vi "Privet.vi"(0 "imya":string) -> ()   [LabVIEW 2016]
uses:
  Global 3.vi
panel:
  in  "?":bool
  in  "поехали":bool
  out "2D Picture":picture
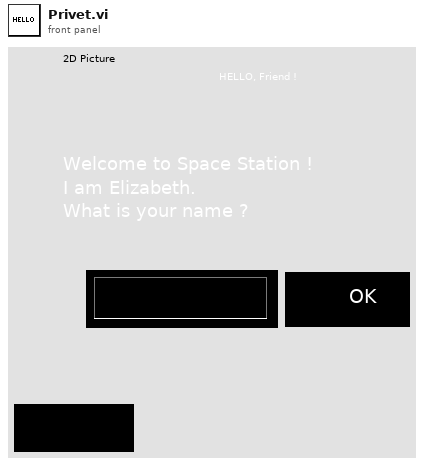
[diagram p1: front panel]
types:
  T1 = enum32{"Invalid", "Standard", "Closed", "Hidden", "Minimized", "Maximized"}
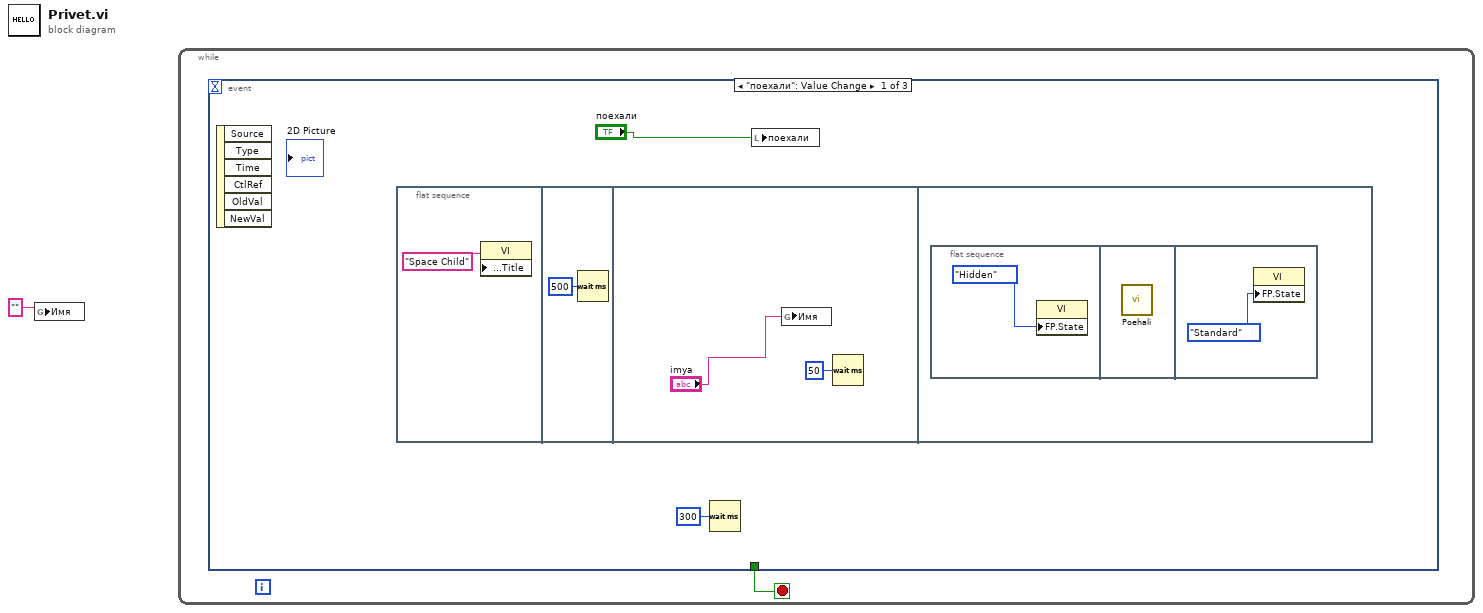
[diagram p0: block diagram]
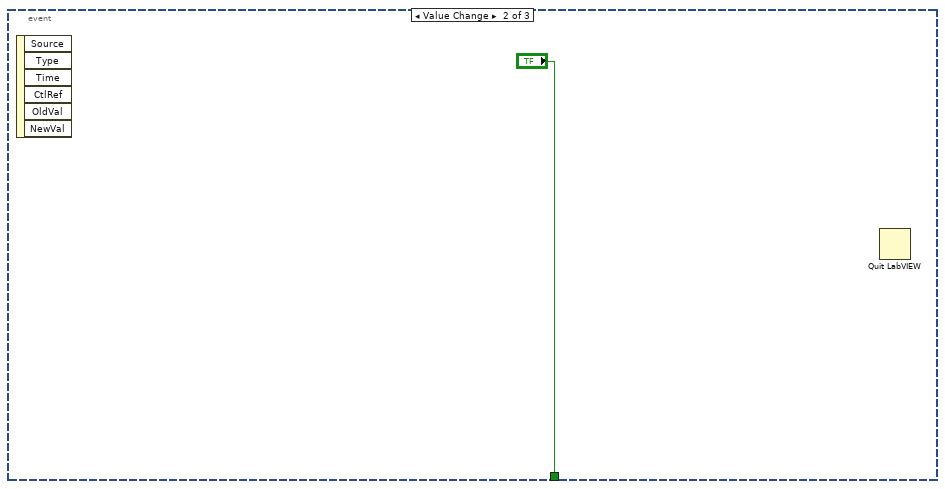
[diagram p2: hidden frame]
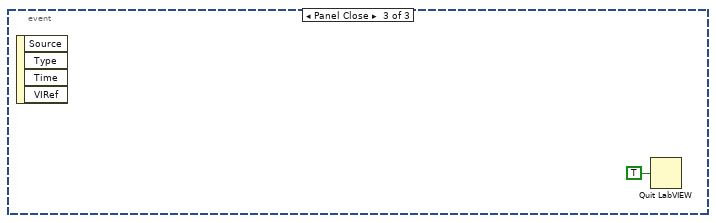
[diagram p3: hidden frame]
diagram:
  n1 = global write "Global 3.vi" "Имя"("") -> ()
  n2 = while {
    stop <- w2 stop-if-true
    n3 = event shown="[0] \"поехали\": Value Change" {
      selector: _ -> [_ _ _]
      dyn-events: _ -> [_ _ _]
      timeout: _ -> [_ _ _]
      tunnel: [_ "?" _] -> w2
      event "поехали": Value Change {
        n4 = event-data() -> ()  [unwired: 1 in, 6 out]
        n5 = flat-sequence {
          frame #0 {
            n6 = property class="VI"("Front Panel.Title"="Space Child" ("Front Panel Window:Title")) -> ()  [unwired: 2 in, 2 out]
          }
          frame #1 {
            n7 = Wait (ms)(milliseconds to wait=u32 500) -> ()  [unwired: 1 out]
          }
          frame #2 {
            n8 = global write "Global 3.vi" "Имя"("imya") -> ()
            n9 = Wait (ms)(milliseconds to wait=u32 50) -> ()  [unwired: 1 out]
          }
          frame #3 {
            n10 = flat-sequence {
              frame #0 {
                n11 = property class="VI"("FP.State"=T1."Hidden" ("Front Panel Window:State")) -> ()  [unwired: 2 in, 2 out]
              }
              frame #1 {
                n12 = call "Poehali.vi"() -> ()  [unwired: 1 out]
              }
              frame #2 {
                n13 = property class="VI"("FP.State"=T1."Standard" ("Front Panel Window:State")) -> ()  [unwired: 2 in, 2 out]
              }
            }
          }
        }
        n14 = Wait (ms)(milliseconds to wait=u32 300) -> ()  [unwired: 1 out]
        n15 = local write "поехали"("поехали") -> ()
      }
      event Value Change {
        n16 = event-data() -> ()  [unwired: 1 in, 6 out]
        n17 = Quit LabVIEW() -> ()  [unwired: 1 in]
      }
      event Panel Close {
        n18 = event-data() -> ()  [unwired: 1 in, 4 out]
        n19 = Quit LabVIEW(quit? (T)=TRUE) -> ()
      }
    }
  }
